vi "Sort Relays.vi"(10 "SwitchActionList":T1 {"RelayAction" items=["CloseRelay"=21, "OpenRelay"=20]}, 11 "Relays":refnum<class "Relay.lvclass">[](array[class])) -> (1 "openList":refnum<class "Relay.lvclass">[](array[class]), 3 "closeList":refnum<class "Relay.lvclass">[](array[class]))   [LabVIEW 2015, in "SLSC Switch.lvlib" / "Switch Action Processor.lvclass"]
uses:
  Switch Action Processor.lvclass
  Relay/Relay.lvclass
  slscsl/SwitchActionsArray.ctl
  slscsl/SwitchAction.ctl
  slscsl/RelayAction.ctl
  slscsl/slscsl.lvclass
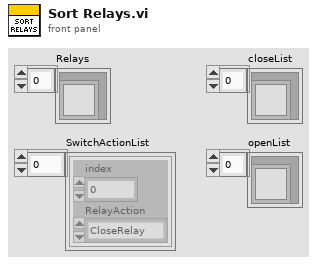
[diagram p1: front panel]
types:
  T1 = typedef "SLSC Switch.lvlib/slscsl.lvclass/SwitchActionsArray.ctl" = T2[]
  T2 = typedef "SLSC Switch.lvlib/slscsl.lvclass/SwitchAction.ctl" = cluster{"index":i32, "RelayAction":T3}
  T3 = typedef "SLSC Switch.lvlib/slscsl.lvclass/RelayAction.ctl" = u32
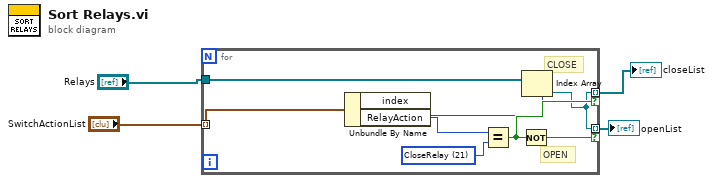
[diagram p0: block diagram]
diagram:
  n1 = for {
    tunnel: "SwitchActionList" -> [w12] mode=indexing
    tunnel: [w5] -> w4 mode=indexing if=w9
    tunnel: [w5] -> w1 mode=indexing if=w8
    tunnel: "Relays" -> [w6]
    w10 = T3 21 items=["CloseRelay"=21, "OpenRelay"=20] ("y")
    # "OPEN"
    # "CLOSE"
    n2 = Unbundle By Name(w12) -> ("index"=w7:i32, "RelayAction"=w11:T3)
    n3 = Equal?(x=w11, y=w10) -> (x = y?=w9:bool)
    n4 = Not(x=w9) -> (.not. x?=w8:bool)
    n5 = Index Array(array=w6, index=w7) -> (element=w5:refnum<class "Relay.lvclass">)
  }
  "closeList" <- w4
  "openList" <- w1
